vi "Update Attributes A.vi"(10 "Attributes":T1) -> (2 "Attributes out":refnum<data-value>)   [LabVIEW 2020, in "jettl.lvlib"]
uses:
  jettl.lvlib
  Actor/Actor.lvclass
  Transport/Transport.lvclass
  Msg/Msg.lvclass
  Msgs.ctl
  Attributes Metadata/Attributes Metadata.lvclass
  Attributes.ctl
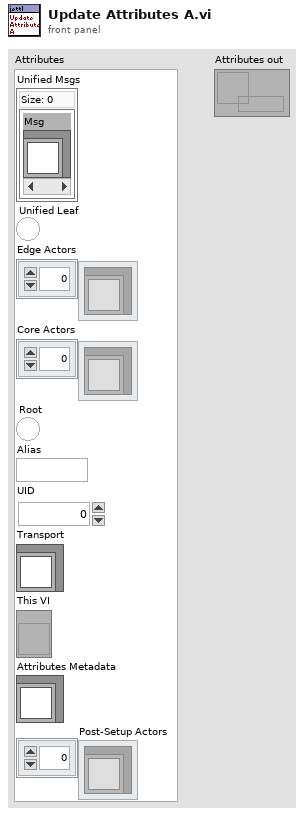
[diagram p1: front panel]
types:
  T1 = typedef "jettl.lvlib/Attributes.ctl" = cluster{"Unified Msgs":T2, "Unified Leaf":bool, "Edge Actors":refnum<class "Actor.lvclass">[], "Core Actors":refnum<class "Actor.lvclass">[], "Root":bool, "Alias":string, "UID":i32, "Transport":refnum<class "Transport.lvclass">, "This VI":refnum<vi>, "Attributes Metadata":refnum<class "Attributes Metadata.lvclass">, "Post-Setup Actors":refnum<class "Actor.lvclass">[]}
  T2 = typedef "jettl.lvlib/Msgs.ctl" = set{refnum<class "Msg.lvclass">}
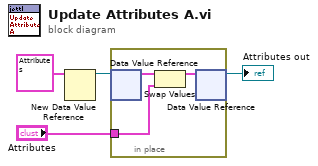
[diagram p0: block diagram]
diagram:
  n1 = New Data Value Reference(data value=T1 {"Unified Msgs"={}, "Unified Leaf"=FALSE, "Edge Actors"=[], "Core Actors"=[], "Root"=FALSE, "Alias"="", "UID"=0, "Transport"=refnum, "This VI"=refnum, "Attributes Metadata"=refnum, "Post-Setup Actors"=[]} ("Attributes")) -> (data value reference=w1:refnum<data-value>)  [unwired: 1 in, 1 out]
  n2 = in-place {
    in-place-border: "Attributes" -> [w7]
    n3 = in-place-dvr #1(w1) -> (w6:T1)  [unwired: 1 out]
    n4 = Swap Values(12:w6, 14:w7) -> (1:w5:T1)  [unwired: 1 in, 1 out]
    n5 = in-place-dvr #1(w5) -> (→"Attributes out":refnum<data-value>)  [unwired: 1 out]
  }
